vi "Distance Drive.vi"(6 "ReInit?":bool, 7 "Distance Tolerance":dbl, 8 "Drive PID Gains":T1, 9 "Y Max Output":dbl, 10 "Y Min Output":dbl, 11 "Distance Target":dbl) -> (0 "Finished":bool, 2 "Y Output":dbl)   [LabVIEW 2017]
uses:
  Common Code/PID Gains Cluster.ctl
  <vilib>/addons/control/pid/pid.llb/PID (DBL).vi
  <vilib>/addons/control/pid/NI_PID_pid.lvlib
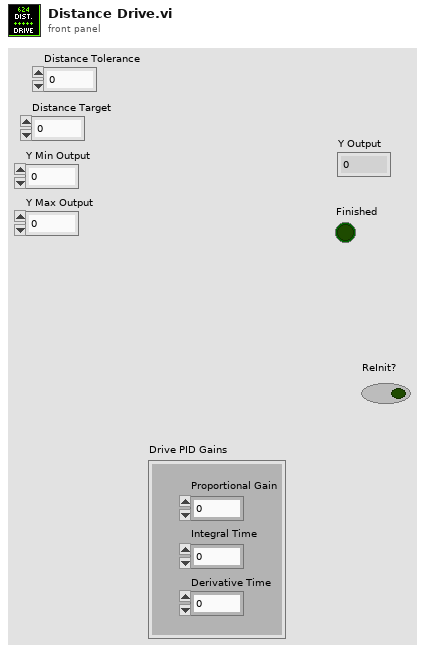
[diagram p1: front panel]
types:
  T1 = typedef "PID Gains Cluster.ctl" = cluster{"Integral Time":dbl, "Proportional Gain":dbl, "Derivative Time":dbl}
  T2 = typedef "Drivetrain Encoder Values.ctl" = cluster{"Left Encoder":cluster{"Distance":dbl, "Speed":dbl, "Tick":dbl}, "Right Encoder":cluster{"Distance":dbl, "Speed":dbl, "Tick":dbl}}
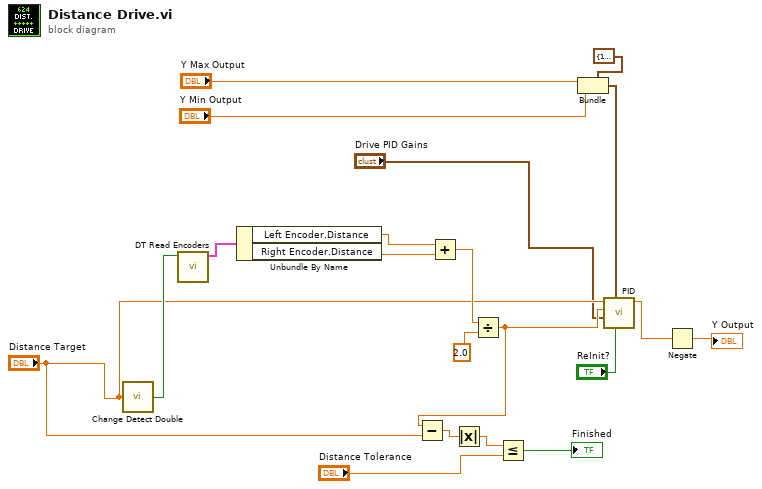
[diagram p0: block diagram]
diagram:
  n1 = call "Change Detect Double.vi"("In"="Distance Target") -> ("Changed?"=w13:bool)
  n2 = call "DT Read Encoders.vi"("Reset Encoders"=w13) -> ("DT Encoder Values"=w4:T2)  [unwired: 10 in]
  n3 = Unbundle By Name(w4) -> ("Left Encoder.Distance"=w3:dbl, "Right Encoder.Distance"=w2:dbl)
  n4 = Add(x=w3, y=w2) -> (x+y=w14:dbl)
  n5 = Divide(x=w14, y=2.0) -> (x/y=w15:dbl)
  n6 = Subtract(x=w15, y="Distance Target") -> (x-y=w11:dbl)
  n7 = Absolute Value(x=w11) -> (abs(x)=w10:dbl)
  n8 = Less Or Equal?(x=w10, y="Distance Tolerance") -> (x <= y?=→"Finished":bool)
  n9 = Bundle(cluster=cluster{dbl, dbl} {100.0, -100.0}, "Y Max Output", "Y Min Output") -> (w19:cluster{dbl, dbl})
  n10 = call-poly <vilib>:"PID.vi"("reinitialize? (F)"="ReInit?", "output range"=w19, "PID gains"="Drive PID Gains", "process variable"=w15, "setpoint"="Distance Target") -> ("output"=w16:dbl)  [unwired: 5 in, 1 out]
  n11 = Negate(x=w16) -> (-x=→"Y Output":dbl)
